vi "BBE数据写入.vi"(7 "初级生产力启用":bool, 8 "错误输入（无错误）":errorcluster, 9 "初级生产力":T1, 10 "data":T2={"时间"=timestamp(0 s since 1904-01-01), "测量模式"="水样测试", "数据类型"="N", "数据标识"="N", "湖面水深"=0.0, "缆绳下放长度"=0.0, "层数"=0, "row"=0, "水温"=0.0, "DO"=0.0, "饱和度"=0.0, "绿藻"=0.0, "蓝藻"=0.0, "硅甲藻"=0.0, "隐藻"=0.0, "黄色物质"=0.0, "总藻"=0.0, "透光率"=0.0, "水深"=0.0, "设置水深"=0.0}, 11 "Tabe Name":string="剖面数据") -> (0 "错误输出":errorcluster)   [LabVIEW 2016, in "main.lvlib"]
uses:
  main.lvlib
panel:
  in  "data 2":cluster{"Fv/Fm":sgl, "PAR":sgl, "GPP":sgl}
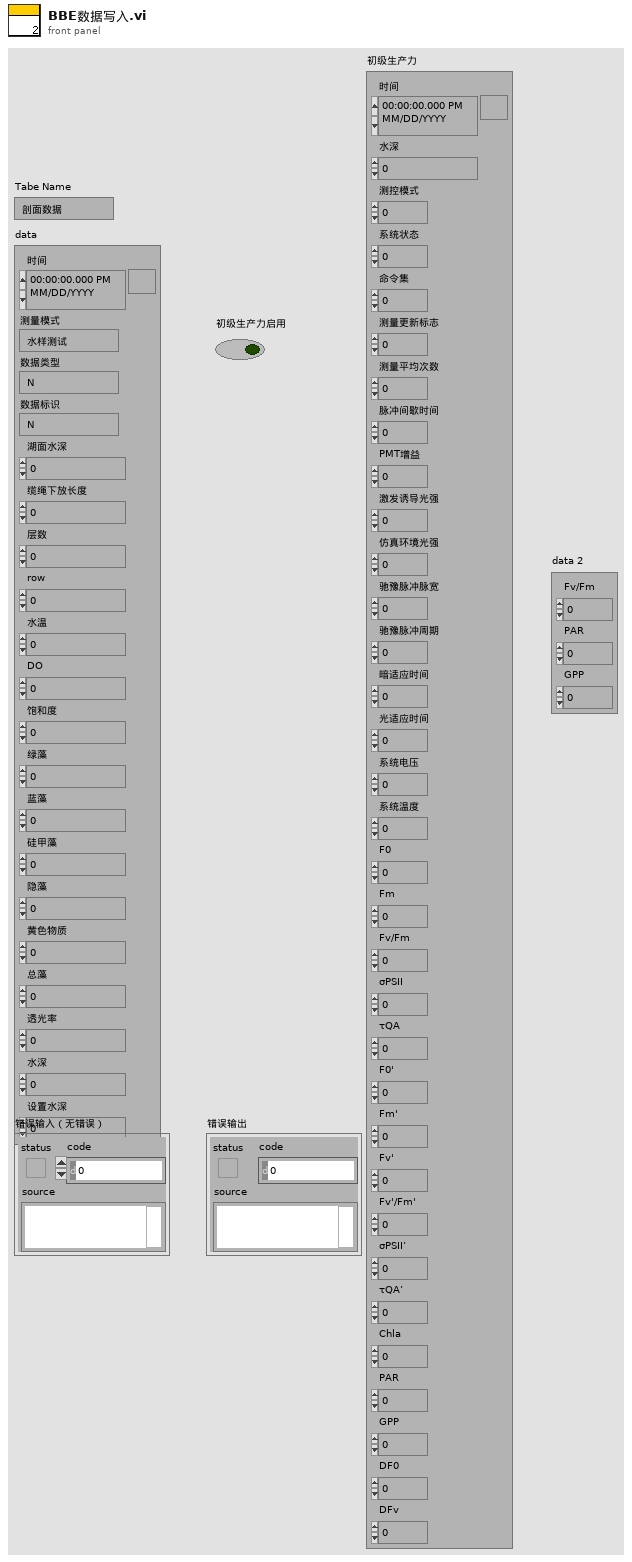
[diagram p1: front panel]
types:
  T1 = cluster{"时间":timestamp, "水深":sgl, "测控模式":u16, "系统状态":u16, "命令集":u16, "测量更新标志":u16, "测量平均次数":u16, "脉冲间歇时间":u16, "PMT增益":u16, "激发诱导光强":u16, "仿真环境光强":u16, "驰豫脉冲脉宽":u16, "驰豫脉冲周期":u16, "暗适应时间":u16, "光适应时间":u16, "系统电压":sgl, "系统温度":sgl, "F0":sgl, "Fm":sgl, "Fv/Fm":sgl, "σPSII":sgl, "τQA":sgl, "F0'":sgl, "Fm'":sgl, "Fv'":sgl, "Fv'/Fm'":sgl, "σPSII’":sgl, "τQA’":sgl, "Chla":sgl, "PAR":sgl, "GPP":sgl, "DF0":sgl, "DFv":sgl}
  T2 = typedef "剖面数据_bbe_NAQDO.ctl" = cluster{"时间":timestamp, "测量模式":string, "数据类型":string, "数据标识":string, "湖面水深":sgl, "缆绳下放长度":sgl, "层数":u16, "row":u16, "水温":sgl, "DO":sgl, "饱和度":sgl, "绿藻":sgl, "蓝藻":sgl, "硅甲藻":sgl, "隐藻":sgl, "黄色物质":sgl, "总藻":sgl, "透光率":sgl, "水深":sgl, "设置水深":sgl}
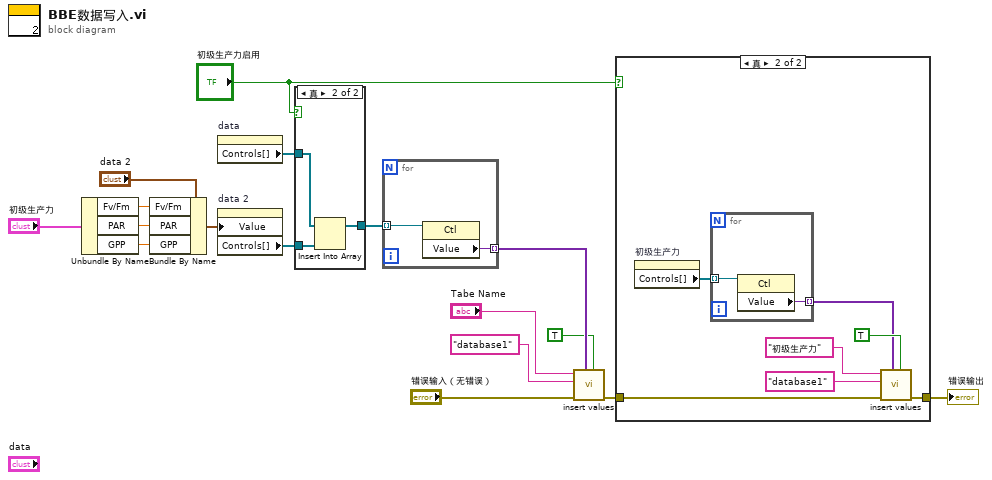
[diagram p0: block diagram]
diagram:
  n1 = Unbundle By Name("初级生产力") -> ("Fv/Fm"=w6:sgl, "PAR"=w5:sgl, "GPP"=w4:sgl)
  n2 = Bundle By Name(cluster="data 2", "Fv/Fm"=w6, "PAR"=w5, "GPP"=w4) -> (w9:cluster{"Fv/Fm":sgl, "PAR":sgl, "GPP":sgl})
  n3 = property on="data" class="Clust (严格)"() -> ("Controls[]"=w12:refnum<vi>[])  [unwired: 2 in, 2 out]
  n4 = property on="data 2" class="Clust (严格)"("Value"=w9) -> ("Controls[]"=w11:refnum<vi>[])  [unwired: 2 in, 2 out]
  n5 = case shown="真" "初级生产力启用" {
    tunnel: w12 -> [w18 w21]
    tunnel: w11 -> [_ w20]
    tunnel: [w18 w19] -> w10
    frame False {
    }
    frame True {
      n6 = Insert Into Array(array=w21, new element=w20) -> (w19:refnum<vi>[])  [unwired: 1 in]
    }
  }
  n7 = for {
    tunnel: w10 -> [w23] mode=indexing
    tunnel: [w22] -> w17 mode=indexing
    n8 = property class="Ctl"(reference=w23) -> ("Value"=w22:variant)  [unwired: 1 in, 2 out]
  }
  n9 = call "insert values.vi"("是否创建唯一键"=TRUE, "data"=w17, "错误输入（无错误）"="错误输入（无错误）", "database"="database1", "Tabe Name"="Tabe Name") -> ("错误输出"=w3:errorcluster)  [unwired: 6 in]
  n10 = case shown="真" "初级生产力启用" {
    tunnel: w3 -> [w24 w27]
    tunnel: [w24 w26] -> w1
    frame False {
    }
    frame True {
      n11 = property on="初级生产力" class="Clust (严格)"() -> ("Controls[]"=w25:refnum<vi>[])  [unwired: 2 in, 2 out]
      n12 = for {
        tunnel: w25 -> [w33] mode=indexing
        tunnel: [w32] -> w29 mode=indexing
        n13 = property class="Ctl"(reference=w33) -> ("Value"=w32:variant)  [unwired: 1 in, 2 out]
      }
      n14 = call "insert values.vi"("是否创建唯一键"=TRUE, "data"=w29, "错误输入（无错误）"=w27, "database"="database1", "Tabe Name"="初级生产力") -> ("错误输出"=w26:errorcluster)  [unwired: 6 in]
    }
  }
  "错误输出" <- w1
